vi "writeToXML.vi"(8 "error in (no error)":errorcluster, 10 "ClassLabel":string, 11 "SetOperatorAccessMode in":refnum<class "SetOperatorAccessMode.lvclass">) -> (0 "error out":errorcluster, 2 "XML out":string, 3 "SetOperatorAccessMode out":refnum<class "SetOperatorAccessMode.lvclass">)   [LabVIEW 2022 SP3, in "TCSDataDefinitions.lvlib" / "TCSCommand.lvlib" / "SetAccessMode.lvlib" / "SetOperatorAccessMode.lvclass"]
uses:
  SetOperatorAccessMode.lvclass
  SetAccessMode/SetAccessMode.lvclass
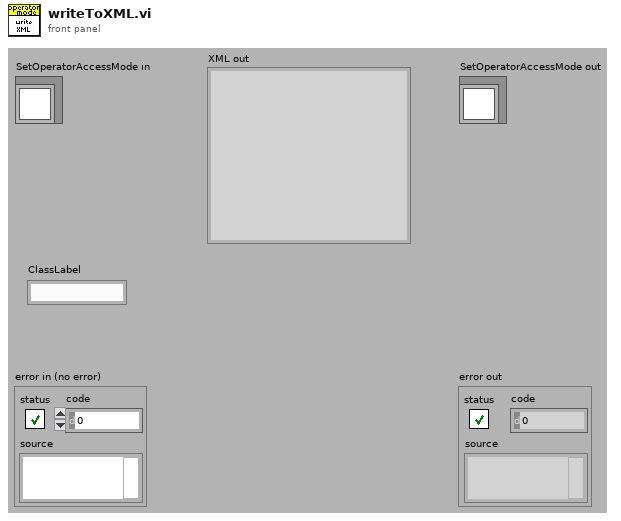
[diagram p1: front panel]
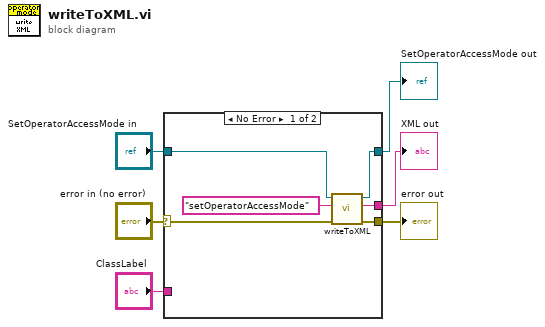
[diagram p0: block diagram]
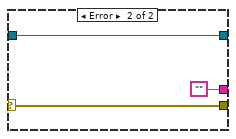
[diagram p2: hidden frame]
diagram:
  n1 = case shown="No Error" "error in (no error)" {
    selector: "error in (no error)" -> [w9 w15]
    tunnel: [w8 w15] -> w5
    tunnel: [w11 w14] -> w3
    tunnel: "SetOperatorAccessMode in" -> [w12 w14]
    tunnel: [w7 ""] -> w2
    tunnel: "ClassLabel" -> [_ _]
    frame No Error {
      n2 = call-parent "writeToXML.vi"("error in (no error)"=w9, "ClassLabel"="setOperatorAccessMode", "SetAccessMode in"=w12) -> ("error out"=w8:errorcluster, "XML out"=w7:string, "SetAccessMode out"=w11:refnum<class "SetOperatorAccessMode.lvclass">)  [unwired: 6 in]
    }
    frame Error {
    }
  }
  "error out" <- w5
  "SetOperatorAccessMode out" <- w3
  "XML out" <- w2
